vi "TenHzDataArray(Global).vi"() -> ()   [LabVIEW 2019]
panel:
  in  "TenHzDataArray":dbl[][](array[numeric])
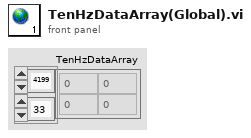
[diagram p1: front panel]
diagram:
